vi "Create_Raw_data_folder.vi"(1 "Folder Name":string="Paul:DispC", 2 "Short_Name":string, 3 "Data Type":string="Colour Calib") -> (0 "Raw Data Folder":path)   [LabVIEW 2014]
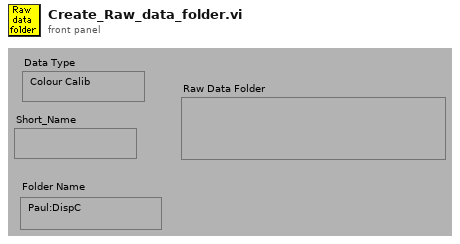
[diagram p1: front panel]
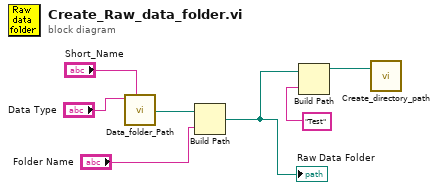
[diagram p0: block diagram]
diagram:
  n1 = call "Data_folder_Path.vi"("Data Type"="Data Type", "Short_Name"="Short_Name") -> ("Data Folder"=w4:path)  [unwired: 4 in]
  n2 = Build Path(base path=w4, name or relative path="Folder Name") -> (appended path=w2:path)
  "Raw Data Folder" <- w2
  n3 = Build Path(base path=w2, name or relative path="Test" ("Substring")) -> (appended path=w6:path)
  n4 = call "Create_directory_path.vi"("Path name"=w6) -> ()  [unwired: 1 in, 2 out]
